vi "NapovedaEKG(subVI).vi"() -> ()   [LabVIEW 2026]
panel:
  in  "Close":bool
  # "1. Před nalepením elektrod se ujistěte, že je kůže v místech, kam budete nalepovat elektrody čistá a pokud možno bez \n    ochlupení. Klidně lze kůži otřít navlhčeným ubrouskem\n2. Vybalte a nalepte na dobrovolníka elektrody podle vámi zvoleného zapojení EKG elektrod. Je doporučen svod II.\n3. Označení elektrod je na PLUX BITalino následující:\n        - černá: záporná elektroda (pro svod II nalepte pod pravou klíční kost)\n        - červená: kladná elektroda (pro svod II nalepte nad levou kyčel)\n        - bílá: referenční elektroda (pro svod II nalepte na pravou kyčel)\n4. Na nalepené elektrody nacvakněte kabely od PLUX BITalina.\n5. Kabel s elektrodami připojte do propojky s nápisem ECG do portu, u kterého není nápis ECG\n6. Do propojky k nápisu ECG zapojte propojovací kabel a jeho druhý konec do portu A3.\n7. Zapněte PLUX BITalino (LED musí pulsovat)\n8. Nastavte parametry pro měření a spusťte jej.\n....."
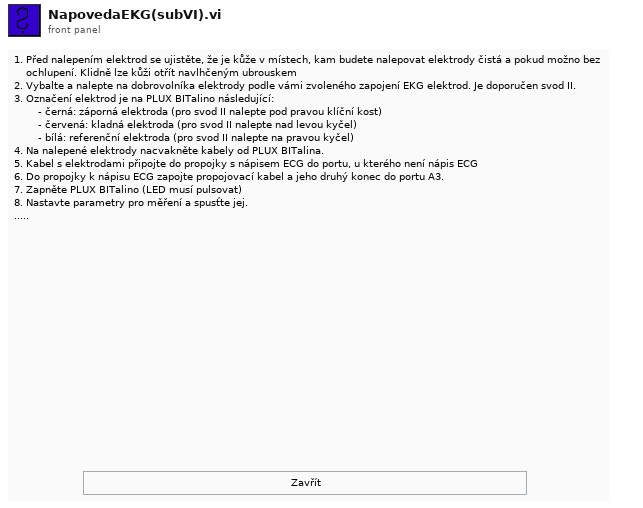
[diagram p1: front panel]
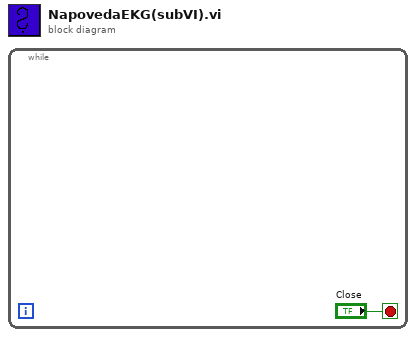
[diagram p0: block diagram]
diagram:
  n1 = while {
    stop <- "Close" stop-if-true
  }
